vi "Subscribe to Group (Name).vi"(7 "Group Type":refnum<class "Group.lvclass">, 8 "error in (no error)":errorcluster, 9 "DataHandler (None)":refnum<class "SubscribedDataHandler.lvclass">, 10 "Group Name":string, 11 "VolatusAPI in":refnum<class "VolatusAPI.lvclass">) -> (0 "error out":errorcluster, 2 "Group":refnum<class "Group.lvclass">, 3 "VolatusAPI out":refnum<class "VolatusAPI.lvclass">)   [LabVIEW 2020, in "Volatus.lvlib" / "VolatusAPI.lvclass"]
uses:
  VolatusAPI.lvclass
  lv-vecto/Vecto/Group/Group.lvclass
  lv-vecto/Vecto/SubscribedDataHandler/SubscribedDataHandler.lvclass
  VolatusAPI.lvclass/VolatusAPI.ctl
  lv-vecto/Vecto/ChannelService/Create Group Abstract.vi
  lv-vecto/Vecto/RemoteDataService/RemoteDataService.lvclass
  VolatusConfig/Node/Node Config.lvclass
  VolatusConfig/Cluster/Cluster Config.lvclass
  VolatusConfig/Group/Group Config.lvclass
  lv-vecto/Vecto/ChannelService/ChannelService.lvclass
  lv-vecto/Vecto/Group Config/Group Config.lvclass
  Event Level.ctl
  Volatus.lvlib
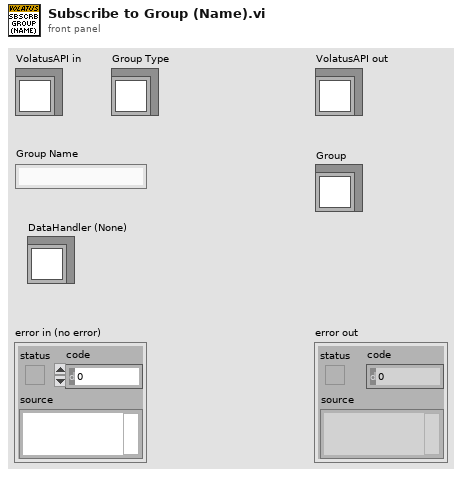
[diagram p1: front panel]
types:
  T1 = typedef "Volatus.lvlib/Event Level.ctl" = enum16{"Debug", "Info", "Warning", "Error"}
  T2 = typedef "VectoConfig.lvlib/Group Info.ctl" = cluster{"System":string, "Cluster":string, "Node":string, "Task":string, "Name":string}
  T3 = typedef "VectoConfig.lvlib/Telemetry Config.ctl" = cluster{"Routing":T4, "Endpoint":T5}
  T4 = typedef "VectoConfig.lvlib/Telemetry Routing.ctl" = enum16{"Multicast", "Unicast"}
  T5 = typedef "VectoConfig.lvlib/Endpoint.ctl" = cluster{"Address":string, "Port":u16}
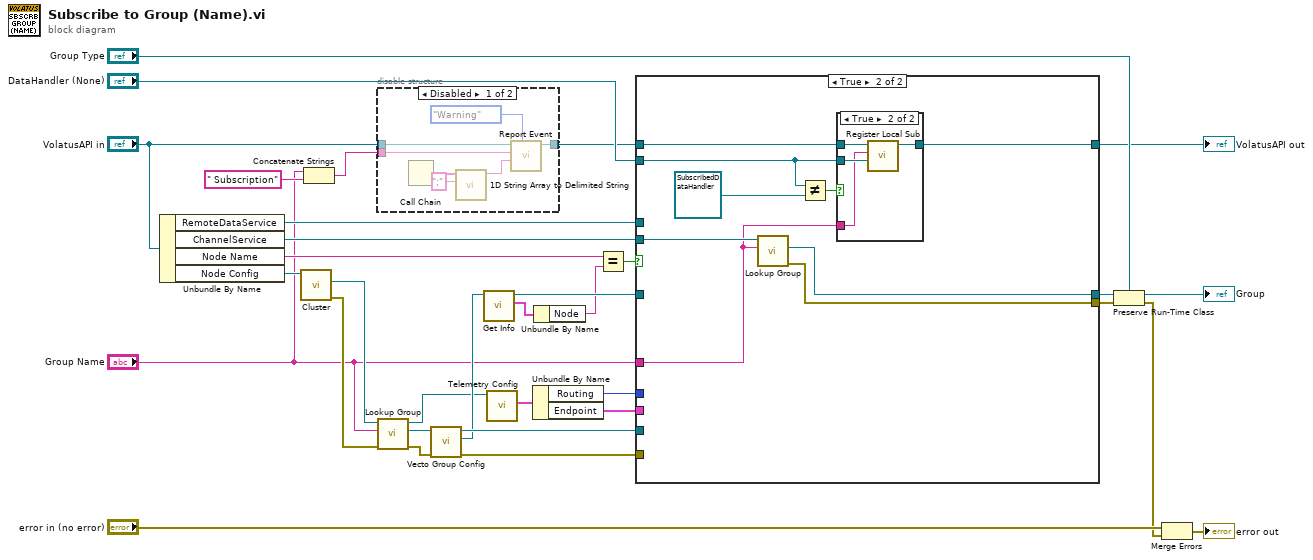
[diagram p0: block diagram]
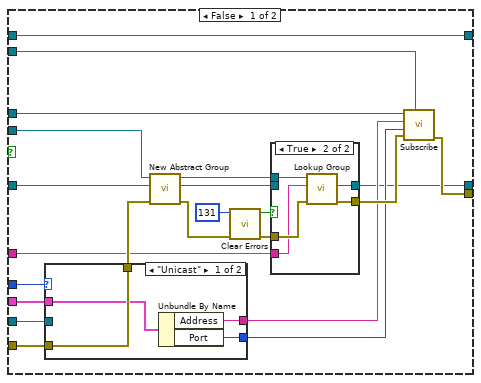
[diagram p3: hidden frame]
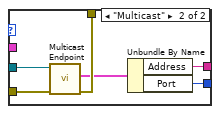
[diagram p4: hidden frame]
diagram:
  n1 = Unbundle By Name("VolatusAPI in") -> ("RemoteDataService"=w30:refnum<class "RemoteDataService.lvclass">, "ChannelService"=w28:refnum<class "ChannelService.lvclass">, "Node Name"=w14:string, "Node Config"=w29:refnum<class "Node Config.lvclass">)
  n2 = call "Cluster.vi"("Node in"=w29) -> ("error out"=w32:errorcluster, "Cluster"=w9:refnum<class "Cluster Config.lvclass">)  [unwired: 8 in, 1 out]
  n3 = Concatenate Strings("Group Name", " Subscription") -> (w1:string)
  n4 = disable-structure shown="Disabled" {
    disable-tunnel: "VolatusAPI in" -> [w40 w41]
    disable-tunnel: [w39 w41] -> w4
    disable-tunnel: w1 -> [w37 _]
    frame Disabled {
      n5 = Call Chain() -> (call chain=w36:string[])
      n6 = call <vilib>:"1D String Array to Delimited String.vi"("delimiter"=";", "string array"=w36) -> ("delimited string"=w34:string)  [unwired: 9 in]
      n7 = call "Report Event.vi"("Level (Info)"=Event_Level."Warning", "Message"=w34, "Context"=w37, "VolatusAPI in"=w40) -> ("VolatusAPI out"=w39:refnum<class "VolatusAPI.lvclass">)  [unwired: 6 in, 1 out]
    }
    frame Enabled {
    }
  }
  n8 = call "Lookup Group.vi"("error in (no error)"=w32, "Group Name"="Group Name", "Cluster in"=w9) -> ("error out"=w26:errorcluster, "Group"=w27:refnum<class "Group Config.lvclass">, "Cluster out"=w8:refnum<class "Cluster Config.lvclass">)  [unwired: 5 in, 1 out]
  n9 = call "Vecto Group Config.vi"("error in (no error)"=w26, "Group in"=w27) -> ("error out"=w25:errorcluster, "Vecto Group Config"=w17:refnum<class "Group Config.lvclass">, "Group out"=w24:refnum<class "Group Config.lvclass">)  [unwired: 7 in]
  n10 = call "Get Info.vi"("Group Config in"=w17) -> ("Info"=w15:T2, "Group Config out"=w16:refnum<class "Group Config.lvclass">)  [unwired: 8 in, 1 out]
  n11 = call "Telemetry Config.vi"("Cluster Config in"=w8) -> ("Telemetry Config"=w7:T3)  [unwired: 8 in, 2 out]
  n12 = Unbundle By Name(w7) -> ("Routing"=w6:T4, "Endpoint"=w5:T5)
  n13 = Unbundle By Name(w15) -> ("Node"=w13:string)
  n14 = Equal?(x=w14, y=w13) -> (x = y?=w12:bool)
  n15 = case shown="True" w12 {
    tunnel: [w62 w84] -> w33
    tunnel: w30 -> [w60 _]
    tunnel: w28 -> [w59 w88]
    tunnel: w25 -> [w56 _]
    tunnel: w24 -> [w55 _]
    tunnel: "Group Name" -> [w48 w82]
    tunnel: [w47 w85] -> w22
    tunnel: "DataHandler (None)" -> [w46 w83]
    tunnel: w16 -> [w45 _]
    tunnel: w4 -> [w44 w86]
    tunnel: [w44 w81] -> w10
    tunnel: w6 -> [w43 _]
    tunnel: w5 -> [w42 _]
    frame False {
      n16 = case shown="\"Unicast\"" w43 {
        tunnel: [w67 w73] -> w61
        tunnel: [w65 w71] -> w58
        tunnel: [w64 w70] -> w57
        tunnel: w56 -> [w67 w69]
        tunnel: w55 -> [_ w68]
        tunnel: w42 -> [w66 _]
        frame "Unicast" {
          n17 = Unbundle By Name(w66) -> ("Address"=w65:string, "Port"=w64:u16)
        }
        frame "Multicast" {
          n18 = call "Multicast Endpoint.vi"("error in (no error)"=w69, "Group in"=w68) -> ("error out"=w73:errorcluster, "Multicast Endpoint"=w72:T5)  [unwired: 7 in, 1 out]
          n19 = Unbundle By Name(w72) -> ("Address"=w71:string, "Port"=w70:u16)
        }
      }
      n20 = call "New Abstract Group.vi"("error in (no error)"=w61, "Group Config"=w45, "ChannelService in"=w59) -> ("error out"=w54:errorcluster, "Group"=w49:refnum<class "Group.lvclass">, "ChannelService out"=w52:refnum<class "ChannelService.lvclass">)  [unwired: 6 in]
      n21 = call <vilib>:"Clear Errors.vi"("error in (no error)"=w54, "specific error code to clear (0: all)"=131) -> ("error out"=w50:errorcluster, "specific error cleared?"=w51:bool)  [unwired: 4 in]
      n22 = case shown="True" w51 {
        tunnel: w52 -> [_ w80]
        tunnel: w50 -> [w75 w79]
        tunnel: w49 -> [w74 _]
        tunnel: w48 -> [_ w78]
        tunnel: [w75 w77] -> w63
        tunnel: [w74 w76] -> w47
        frame False {
        }
        frame True {
          n23 = call "Lookup Group.vi"("error in (no error)"=w79, "Group Name"=w78, "ChannelService in"=w80) -> ("error out"=w77:errorcluster, "Group"=w76:refnum<class "Group.lvclass">)  [unwired: 6 in, 1 out]
        }
      }
      n24 = call "Subscribe.vi"("DataHandler (None)"=w46, "error in (no error)"=w63, "Port"=w57, "Address"=w58, "RemoteDataService in"=w60) -> ("error out"=w62:errorcluster)  [unwired: 5 in, 1 out]
    }
    frame True {
      n25 = call "Lookup Group.vi"("Group Name"=w82, "ChannelService in"=w88) -> ("error out"=w84:errorcluster, "Group"=w85:refnum<class "Group.lvclass">)  [unwired: 7 in, 1 out]
      n26 = Not Equal?(x=w83, y=refnum<class "SubscribedDataHandler.lvclass"> refnum) -> (x != y?=w87:bool)
      n27 = case shown="True" w87 {
        tunnel: w86 -> [w90 w94]
        tunnel: w83 -> [_ w93]
        tunnel: w82 -> [_ w92]
        tunnel: [w90 w91] -> w81
        frame False {
        }
        frame True {
          n28 = call "Register Local Sub.vi"("Data Handler"=w93, "Group Name"=w92, "VolatusAPI in"=w94) -> ("VolatusAPI out"=w91:refnum<class "VolatusAPI.lvclass">)  [unwired: 7 in, 1 out]
        }
      }
    }
  }
  "VolatusAPI out" <- w10
  n29 = Preserve Run-Time Class(object in=w22, error in=w33, 2:"Group Type") -> (object out=→"Group":refnum<class "Group.lvclass">, error out=w19:errorcluster)
  n30 = Merge Errors("error in (no error)", w19) -> (→"error out":errorcluster)
